vi "Power On (4-port).vi"(0 "Power Port 1 in":refnum<visa-resource-name>="COM12", 5 "Power Port 2 in":refnum<visa-resource-name>="COM12", 9 "On/Off":enum16{"Power Off", "Power On"}(ring), 11 "error in (no error)":errorcluster, 12 "Valid":bool[](array[boolean])) -> (4 "Power Port 1 out":refnum<visa-resource-name>="COM12", 6 "Power Port 2 out":refnum<visa-resource-name>="COM12", 15 "error out":errorcluster)   [LabVIEW 2010]
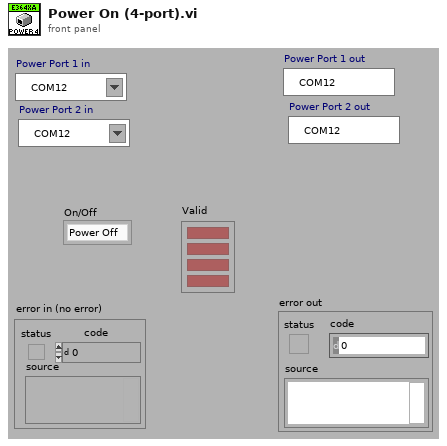
[diagram p1: front panel]
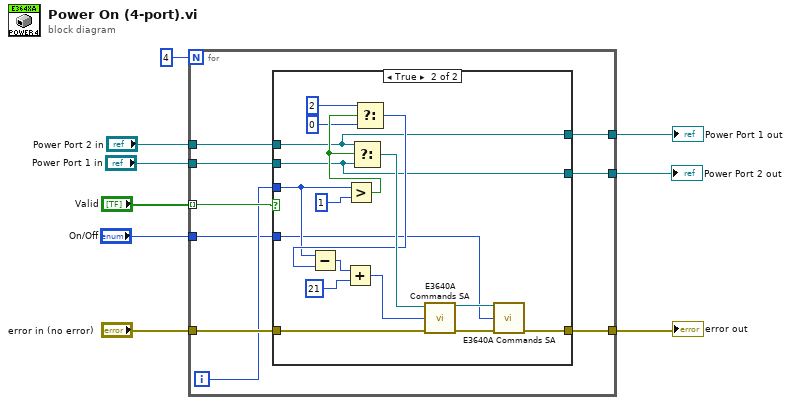
[diagram p0: block diagram]
diagram:
  n1 = for {
    N: 4 -> [_]
    tunnel: "error in (no error)" -> [w18]
    tunnel: "Power Port 1 in" -> [w17]
    tunnel: "Power Port 2 in" -> [w16]
    tunnel: "Valid" -> [w15] mode=indexing
    tunnel: [w13] -> w4
    tunnel: [w12] -> w3
    tunnel: [w11] -> w2
    tunnel: "On/Off" -> [w10]
    i -> [w14]
    n2 = case shown="True" w15 {
      tunnel: w18 -> [w19 w38]
      tunnel: w17 -> [w20 w26]
      tunnel: w16 -> [w21 w27]
      tunnel: w14 -> [_ w28]
      tunnel: [w21 w27] -> w13
      tunnel: [w20 w26] -> w12
      tunnel: [w19 w25] -> w11
      tunnel: w10 -> [_ w22]
      frame False {
      }
      frame True {
        n3 = Greater?(x=w28, y=1) -> (0:w33:bool)
        n4 = Select(t=w27, s=w33, f=w26) -> (s? t:f=w34:refnum<visa-resource-name>)
        n5 = Select(t=2, s=w33, f=0) -> (s? t:f=w29:i32)
        n6 = Subtract(x=w28, y=w29) -> (x-y=w30:i32)
        n7 = Add(x=w30, y=21) -> (x+y=w37:i32)
        n8 = call "E3640A Commands SA.vi"("VISA session"=w34, "Command"=w37, "error in (no error)"=w38) -> ("VISA session out"=w23:refnum<visa-resource-name>, "error out"=w24:errorcluster)  [unwired: 7 in, 4 out]
        n9 = call "E3640A Commands SA.vi"("VISA session"=w23, "Command"=w22, "error in (no error)"=w24) -> ("error out"=w25:errorcluster)  [unwired: 7 in, 5 out]
      }
    }
  }
  "error out" <- w2
  "Power Port 1 out" <- w4
  "Power Port 2 out" <- w3
